vi "综合生物毒性写数据库.vi"(8 "错误输入（无错误）":errorcluster, 11 "综合生物毒性":T2={"时间"=timestamp(0 s since 1904-01-01), "水样测量结果"=0.0, "质控测量结果"=0.0, "R0"=0, "S0"=0, "Rt"=0, "St"=0, "CF"=0.0, "测量仓温度"=0.0, "培养仓温度"=0.0, "试剂余量"=0.0, "仪器状态"="", "空白结果"=0.0, "启动测量"=enum."启动水样测量", "停止测量"=FALSE}) -> (0 "错误输出":errorcluster)   [LabVIEW 2016, in "综合生物毒性.lvlib"]
panel:
  in  "Tabe Name":string="综合生物毒性"
  out "data":T1
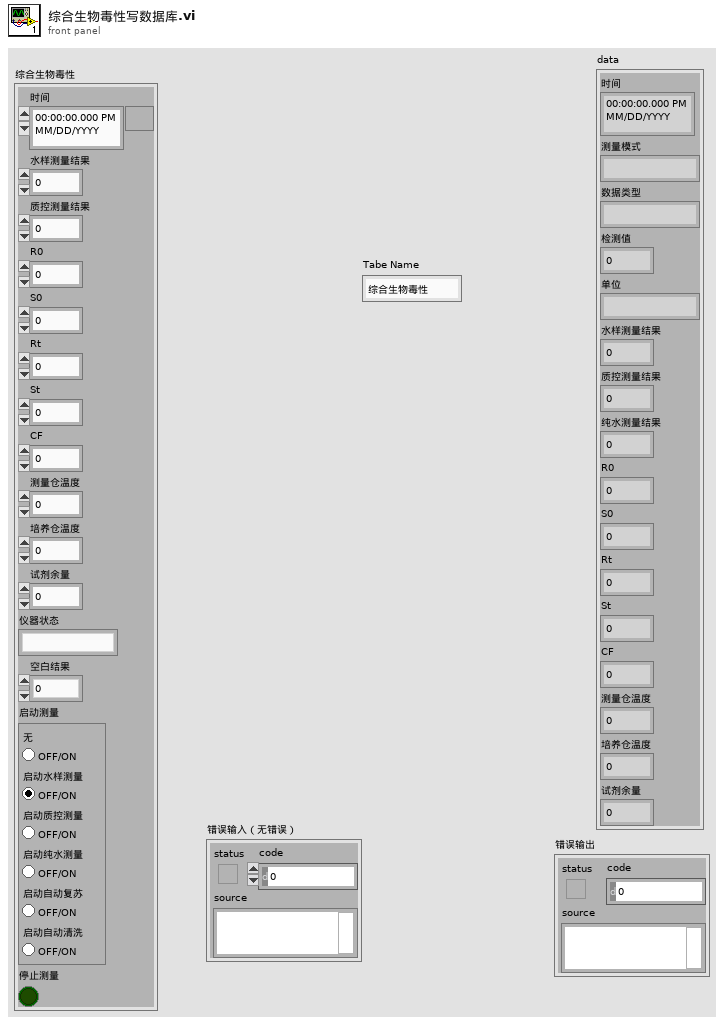
[diagram p1: front panel]
types:
  T1 = cluster{"时间":timestamp, "测量模式":string, "数据类型":string, "检测值":dbl, "单位":string, "水样测量结果":sgl, "质控测量结果":sgl, "纯水测量结果":sgl, "R0":i32, "S0":i32, "Rt":i32, "St":i32, "CF":sgl, "测量仓温度":sgl, "培养仓温度":sgl, "试剂余量":sgl}
  T2 = cluster{"时间":timestamp, "水样测量结果":sgl, "质控测量结果":sgl, "R0":i32, "S0":i32, "Rt":i32, "St":i32, "CF":sgl, "测量仓温度":sgl, "培养仓温度":sgl, "试剂余量":sgl, "仪器状态":string, "空白结果":dbl, "启动测量":enum32{"无", "启动水样测量", "启动质控测量", "启动纯水测量", "启动自动复苏", "启动自动清洗"}, "停止测量":bool}
  T3 = cluster{"启动时间":timestamp, "测量模式":string, "数据类型":string, "空白结果":dbl, "单位":string, "水样测量结果":sgl, "质控测量结果":sgl, "空白结果":dbl, "R0":i32, "S0":i32, "Rt":i32, "St":i32, "CF":sgl, "测量仓温度":sgl, "培养仓温度":sgl, "试剂余量":sgl}
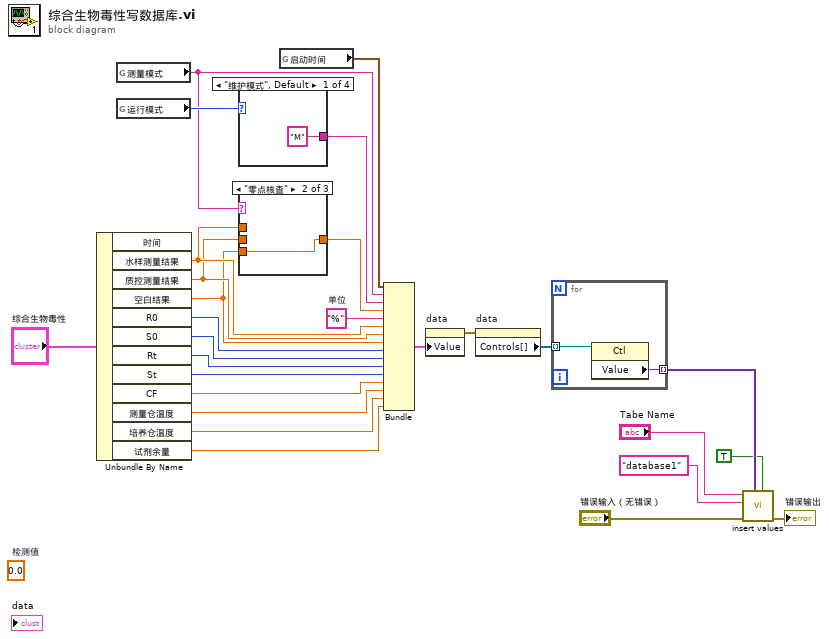
[diagram p0: block diagram]
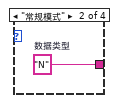
[diagram p4: hidden frame]
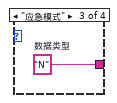
[diagram p5: hidden frame]
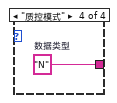
[diagram p6: hidden frame]
diagram:
  (unwired) 0.0  # 检测值
  w25 = "%"  # 单位
  n1 = Unbundle By Name("综合生物毒性") -> ("水样测量结果"=w5:sgl, "质控测量结果"=w4:sgl, "空白结果"=w1:dbl, "R0"=w24:i32, "S0"=w23:i32, "Rt"=w22:i32, "St"=w21:i32, "CF"=w20:sgl, "测量仓温度"=w19:sgl, "培养仓温度"=w18:sgl, "试剂余量"=w17:sgl)  [unwired: 1 out]
  n2 = global read "全局_综合生物毒性.vi" "测量模式"() -> (w6:string)
  n3 = global read "系统设置全局变量.vi" "运行模式"() -> (w7:enum16{"维护模式", "常规模式", "应急模式", "质控模式"})
  n4 = case shown="\"维护模式\", Default" w7 {
    tunnel: ["M" ("数据类型") w29 w30 w31] -> w26
    frame "维护模式", Default {
    }
    frame "常规模式" {
      w29 = "N"  # 数据类型
    }
    frame "应急模式" {
      w30 = "N"  # 数据类型
    }
    frame "质控模式" {
      w31 = "N"  # 数据类型
    }
  }
  n5 = case shown="\"零点核查\"" w6 {
    tunnel: w5 -> [_ _ w34]
    tunnel: [w32 w33 w34] -> w3
    tunnel: w4 -> [w32 _ _]
    tunnel: w1 -> [_ w33 _]
    frame "跨度核查", Default {
    }
    frame "零点核查" {
    }
    frame "水样测试" {
    }
  }
  n6 = global read "全局_综合生物毒性.vi" "启动时间"() -> (w2:timestamp)
  n7 = Bundle("启动时间"=w2, "测量模式"=w6, "数据类型"=w26, "空白结果"=w3, "单位"=w25, "水样测量结果"=w5, "质控测量结果"=w4, "空白结果"=w1, "R0"=w24, "S0"=w23, "Rt"=w22, "St"=w21, "CF"=w20, "测量仓温度"=w19, "培养仓温度"=w18, "试剂余量"=w17) -> (w16:T3)  [unwired: 1 in]
  n8 = property on="data" class="Clust (strict)"("Value"=w16) -> (error out=w8:errorcluster)  [unwired: 2 in, 1 out]
  n9 = property on="data" class="Clust (strict)"(error in=w8) -> ("Controls[]"=w15:refnum<vi>[])  [unwired: 1 in, 2 out]
  n10 = for {
    tunnel: w15 -> [w36] mode=indexing
    tunnel: [w35] -> w14 mode=indexing
    n11 = property class="Ctl"(reference=w36) -> ("Value"=w35:variant)  [unwired: 1 in, 2 out]
  }
  n12 = call "insert values.vi"("是否创建唯一键"=TRUE, "data"=w14, "错误输入（无错误）"="错误输入（无错误）", "database"="database1", "Tabe Name"="Tabe Name") -> ("错误输出"=→"错误输出":errorcluster)  [unwired: 6 in]
